vi "Commands_Update_Erase_JLINK.vi"(0 "Action":enum16{"Erase", "Erase and upload", "Upload"}(ring)=enum."Erase and upload", 1 "Button status":refnum<vi>, 5 "user name":string, 7 "Config Device":T1={"Connection type"="FINE", "speed"="1000", "select device"="R5F52317", "PASSWORD"=""}) -> (4 "command_jlink":string)   [LabVIEW 2023]
uses:
  controls/Config_Devices.ctl
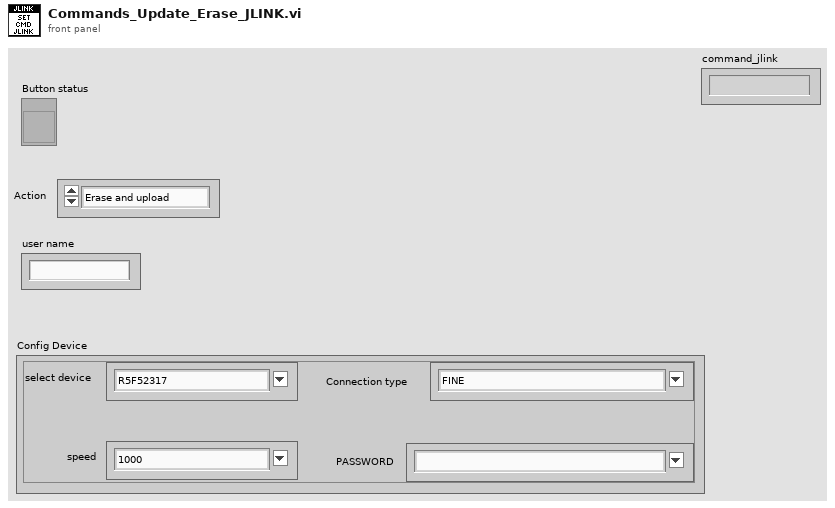
[diagram p1: front panel]
types:
  T1 = typedef "Config_Devices.ctl" = cluster{"Connection type":string, "speed":string, "select device":string, "PASSWORD":string}
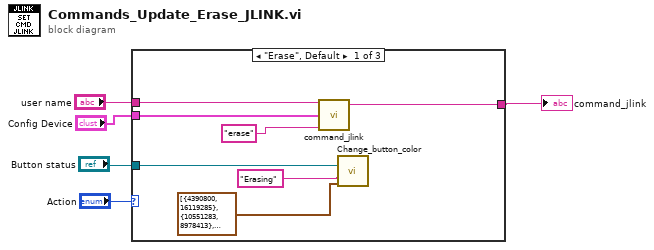
[diagram p0: block diagram]
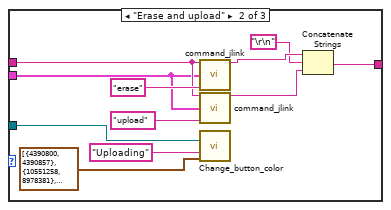
[diagram p2: hidden frame]
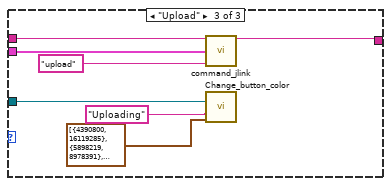
[diagram p3: hidden frame]
diagram:
  n1 = case shown="\"Erase\", Default" "Action" {
    tunnel: "user name" -> [w12 w22 w30]
    tunnel: [w10 w20 w28] -> w1
    tunnel: "Config Device" -> [w9 w16 w27]
    tunnel: "Button status" -> [w8 w15 w26]
    frame "Erase", Default {
      n2 = call "command_jlink.vi"("user"=w12, "Config Device"=w9, "uploader_erase?"="erase") -> ("command_jlink"=w10:string)  [unwired: 12 in]
      n3 = call "Change_button_color.vi"("Button"=w8, "Text"="Erasing", "Colors [4]"=cluster{u32, u32}[] [{4390800, 16119285}, {10551283, 8978413}, {10551283, 10551283}, {65511, 16770137}]) -> ()  [unwired: 13 in]
    }
    frame "Erase and upload" {
      n4 = call "command_jlink.vi"("user"=w22, "Config Device"=w16, "uploader_erase?"="erase") -> ("command_jlink"=w19:string)  [unwired: 12 in]
      n5 = call "command_jlink.vi"("user"=w22, "Config Device"=w16, "uploader_erase?"="upload") -> ("command_jlink"=w17:string)  [unwired: 12 in]
      n6 = call "Change_button_color.vi"("Button"=w15, "Text"="Uploading", "Colors [4]"=cluster{u32, u32}[] [{4390800, 4390857}, {10551258, 8978381}, {10551283, 10551283}, {65511, 16770137}]) -> ()  [unwired: 13 in]
      n7 = Concatenate Strings(w19, "\r\n", w17) -> (w20:string)
    }
    frame "Upload" {
      n8 = call "command_jlink.vi"("user"=w30, "Config Device"=w27, "uploader_erase?"="upload") -> ("command_jlink"=w28:string)  [unwired: 12 in]
      n9 = call "Change_button_color.vi"("Button"=w26, "Text"="Uploading", "Colors [4]"=cluster{u32, u32}[] [{4390800, 16119285}, {5898219, 8978391}, {10551283, 10551283}, {65511, 16770137}]) -> ()  [unwired: 13 in]
    }
  }
  "command_jlink" <- w1
